vi "cw_5_6_v2.vi"() -> ()   [LabVIEW 2022 SP3]
uses:
  c880fe75-26bb-46aa-bcd6-47c0da88fdad.vi
  <vilib>/Comparison/Less/Less Functor/Less Functor.lvclass
panel:
  out "sorted array":i32[](array[numeric])
  out "Array":i32[](array[numeric])
  out "XY Graph":cluster{i32[], dbl[]}(graph)
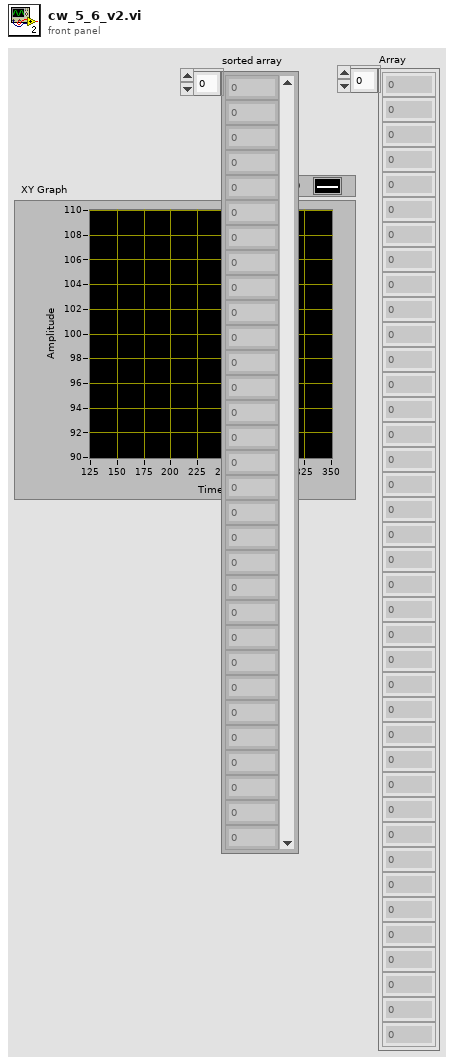
[diagram p1: front panel]
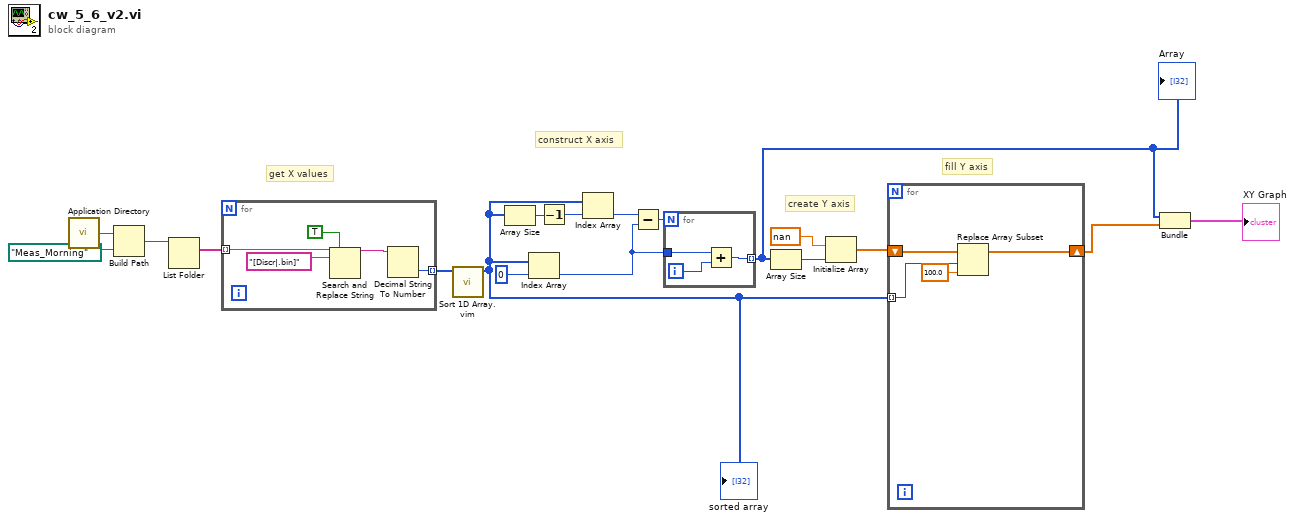
[diagram p0: block diagram]
diagram:
  # "fill Y axis"
  # "get X values"
  # "create Y axis"
  # "construct X axis"
  n1 = call <vilib>:"Application Directory.vi"() -> ("Application Directory"=w18:path)
  n2 = Build Path(base path=w18, name or relative path=path "Meas_Morning") -> (appended path=w16:path)
  n3 = List Folder(path=w16) -> (filenames=w15:string[])  [unwired: 3 in, 3 out]
  n4 = for {
    tunnel: w15 -> [w23] mode=indexing
    tunnel: [w19] -> w14 mode=indexing
    n5 = Search and Replace String(replace all?=TRUE ("replace all? (F)"), input string=w23, search string="[Discr|.bin]") -> (result string=w20:string)  [unwired: 5 in, 3 out]
    n6 = Decimal String To Number(string=w20) -> (number=w19:i32)  [unwired: 2 in, 1 out]
  }
  n7 = call "Sort 1D Array.vim"("unsorted array"=w14) -> ("sorted array"=w6:i32[])  [unwired: 10 in]
  "sorted array" <- w6
  n8 = Array Size(array=w6) -> (size(s)=w12:i32)
  n9 = Index Array(array=w6, index=0) -> (element=w4:i32)
  n10 = Decrement(x=w12) -> (x-1=w11:i32)
  n11 = Index Array(array=w6, index=w11) -> (element=w5:i32)
  n12 = Subtract(x=w5, y=w4) -> (x-y=w10:i32)
  n13 = for {
    N: w10 -> [_]
    tunnel: w4 -> [w25]
    tunnel: [w24] -> w2 mode=indexing
    i -> [w26]
    n14 = Add(x=w25, y=w26) -> (x+y=w24:i32)
  }
  "Array" <- w2
  n15 = Array Size(array=w2) -> (size(s)=w8:i32)
  n16 = Initialize Array(nan, w8) -> (w7:dbl[])
  n17 = for {
    shift-right: [w29] -> w3
    shift-left: w7 -> [w30]
    tunnel: w6 -> [w28] mode=indexing
    n18 = Replace Array Subset(array=w30, new element=100.0 ("new element/subarray"), index=w28) -> (w29:dbl[])
  }
  n19 = Bundle(w2, w3) -> (→"XY Graph":cluster{i32[], dbl[]})  [unwired: 1 in]
